vi "VCS Set Position Compare Parameter.vi"(0 "axis in":cluster{"keyHandle":u32, "nodeId":u16}={"keyHandle"=0, "nodeId"=1}, 7 "position compare parameter":T1 {"operationalMode" items=["single position mode", "position sequence mode"]; "intervalMode" items=["negative direction to reference position", "positive direction to reference position", "positive and negative direction to reference position"]; "directionDependency" items=["negative motor direction", "positive motor direction", "both motor direction"]}, 11 "error in (no error)":errorcluster) -> (4 "axis out":cluster{"keyHandle":u32, "nodeId":u16}={"keyHandle"=0, "nodeId"=1}, 15 "error out":errorcluster)   [LabVIEW 2017, in "maxonEPOS.lvlib"]
doc: "<B>VCS_SetPositionCompareParameter</B> writes all parameters for position compare."
uses:
  Examples/maxonEPOS.lvlib
  SSI_Tool/InstrumentsInterfaces/Motordriver/maxon EPOS/Resources/EposCmd.dll
  SSI_Tool/InstrumentsInterfaces/Motordriver/maxon EPOS/Resources/EposCmd64.dll
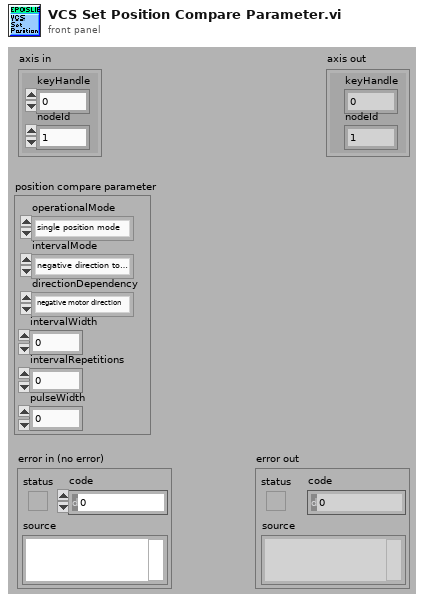
[diagram p1: front panel]
types:
  T1 = cluster{"operationalMode":u8, "intervalMode":u8, "directionDependency":u8, "intervalWidth":u16, "intervalRepetitions":u16, "pulseWidth":u16}
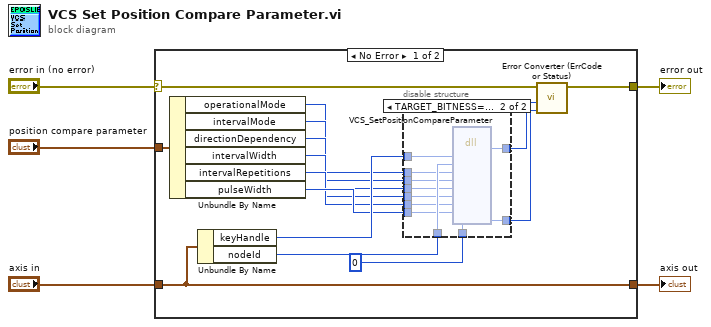
[diagram p0: block diagram]
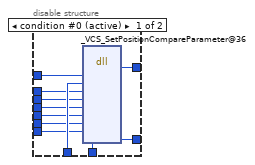
[diagram p2: hidden frame]
diagram:
  n1 = case shown="No Error" "error in (no error)" {
    selector: "error in (no error)" -> [w18 w43]
    tunnel: "axis in" -> [w20 w44]
    tunnel: [w20 w44] -> w4
    tunnel: [w19 w43] -> w3
    tunnel: "position compare parameter" -> [w13 _]
    frame No Error {
      n2 = Unbundle By Name(w13) -> ("operationalMode"=w7:u8, "intervalMode"=w8:u8, "directionDependency"=w9:u8, "intervalWidth"=w10:u16, "intervalRepetitions"=w11:u16, "pulseWidth"=w12:u16)
      n3 = Unbundle By Name(w20) -> ("keyHandle"=w15:u32, "nodeId"=w16:u16)
      n4 = disable-structure shown="TARGET_BITNESS==64" {
        disable-tunnel: u32 0 ("pErrorCode") -> [w31 w42]
        disable-tunnel: w16 -> [w30 w41]
        disable-tunnel: w15 -> [w29 w40]
        disable-tunnel: [w28 w39] -> w14
        disable-tunnel: w12 -> [w27 w38]
        disable-tunnel: w11 -> [w26 w37]
        disable-tunnel: w10 -> [w25 w36]
        disable-tunnel: w9 -> [w24 w35]
        disable-tunnel: w8 -> [w23 w34]
        disable-tunnel: w7 -> [w22 w33]
        disable-tunnel: [w21 w32] -> w6
        frame condition #0 (active) {
          n5 = dll-call lib="C:/workspace/project/scancon/sw/SSI_Tool/InstrumentsInterfaces/Motordriver/maxon EPOS/Resources/EposCmd.*" fn="_VCS_SetPositionCompareParameter@36"("KeyHandle"=w29, "NodeId"=w30, "OperationalMode"=w22, "IntervalMode"=w23, "DirectionDependency"=w24, "IntervalWidth"=w25, "IntervalRepetitions"=w26, "PulseWidth"=w27, "pErrorCode"=w31) -> (w21:i32, "pErrorCode"=w28:u32)  [unwired: 11 in, 2 out]
        }
        frame condition #1 {
          n6 = dll-call lib="C:/setup/Resources/EposCmd64.dll" fn="VCS_SetPositionCompareParameter" ("EposCmd.dll:_VCS_SetPositionCompareParameter@36")("KeyHandle"=w40, "NodeId"=w41, "OperationalMode"=w33, "IntervalMode"=w34, "DirectionDependency"=w35, "IntervalWidth"=w36, "IntervalRepetitions"=w37, "PulseWidth"=w38, "pErrorCode"=w42) -> ("Rückgabetyp"=w32:i32, "pErrorCode"=w39:u32)  [unwired: 11 in, 2 out]
        }
      }
      n7 = call "Error Converter (ErrCode or Status).vi"("error code"=w14, "return type"=w6, "error in (no error)"=w18) -> ("error out"=w19:errorcluster)  [unwired: 7 in]
    }
    frame Error {
    }
  }
  "error out" <- w3
  "axis out" <- w4
